vi "Model Initial Values - Get Number of Inports.vi"(8 "error in (no error)":errorcluster, 11 "ID in":T1 format="%.0x") -> (0 "error out":errorcluster, 1 "GetInportTime":u32, 2 "size(s)":i32, 3 "ID out":T1 format="%.0x", 4 "Numeric":i32)   [LabVIEW 2011, in "Model Initial Values Custom Device.lvlib"]
uses:
  Model Initial Values Custom Device.lvlib
  NationalInstruments.VeriStand.SystemDefinitionAPI
  <vilib>/NI Veristand/Custom Device Offline API/Custom Device Offline API.lvlib
  <vilib>/NI Veristand/Custom Device API/Custom Device Item Ref.ctl
  <vilib>/NI Veristand/Custom Device API/Custom Device API.lvlib
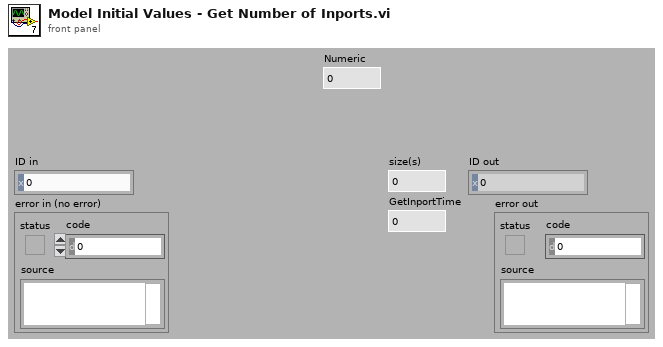
[diagram p1: front panel]
types:
  T1 = typedef "Custom Device API.lvlib/Custom Device Item Ref.ctl" = u64
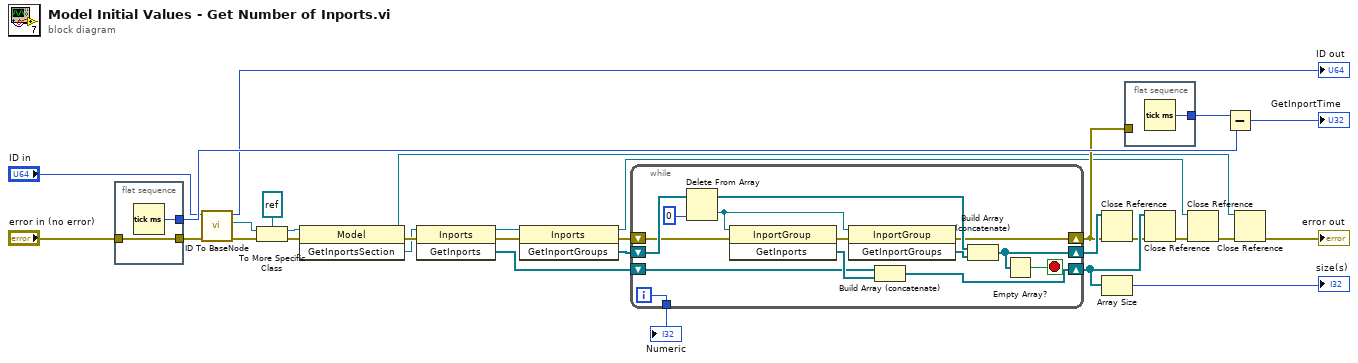
[diagram p0: block diagram]
diagram:
  n1 = flat-sequence {
    tunnel: [w32] -> w23
    tunnel: "error in (no error)" -> [w31]
    tunnel: [w31] -> w16
    frame #0 {
      n2 = Tick Count (ms)() -> (millisecond timer value=w32:u32)
    }
  }
  n3 = call <vilib>:"ID To BaseNode.vi"("error in (no error)"=w16, "ID in"="ID in") -> ("error out"=w28:errorcluster, "BaseNode"=w30:refnum<k24>, "ID out"=→"ID out":u64)  [unwired: 7 in]
  n4 = To More Specific Class(target class=refnum<k24> refnum ("BaseNodeType"), reference=w30, error in=w28) -> (specific class reference=w26:refnum<k24>, error out=w18:errorcluster)
  n5 = invoke class="Model" method="GetInportsSection"(reference=w26, error in=w18) -> (reference out=w2:refnum<k24>, error out=w25:errorcluster, "GetInportsSection"=w15:refnum<k24>)  [unwired: 1 in]
  n6 = invoke class="Inports" method="GetInports"(reference=w15, error in=w25) -> (reference out=w6:refnum<k24>, error out=w12:errorcluster, "GetInports"=w13:refnum<k24>[])  [unwired: 1 in]
  n7 = invoke class="Inports" method="GetInportGroups"(reference=w6, error in=w12) -> (reference out=w5:refnum<k24>, error out=w11:errorcluster, "GetInportGroups"=w14:refnum<k24>[])  [unwired: 1 in]
  n8 = while {
    shift-right: [w37] -> w9
    shift-left: w14 -> [w46]
    shift-right: [w40] -> w10
    shift-left: w13 -> [w39]
    shift-right: [w34] -> w7
    shift-left: w11 -> [w36]
    tunnel: [w33] -> w1
    i -> [w33]
    stop <- w38 stop-if-true
    n9 = Delete From Array(array=w46, index=0) -> (deleted portion=w42:refnum<k24>, array with subset deleted=w44:refnum<k24>[])  [unwired: 1 in]
    n10 = invoke class="InportGroup" method="GetInports"(reference=w42, error in=w36) -> (error out=w35:errorcluster, "GetInports"=w41:refnum<k24>[])  [unwired: 1 in, 1 out]
    n11 = invoke class="InportGroup" method="GetInportGroups"(reference=w42, error in=w35) -> (error out=w34:errorcluster, "GetInportGroups"=w43:refnum<k24>[])  [unwired: 1 in, 1 out]
    n12 = Build Array (concatenate)(w39, w41) -> (w40:refnum<k24>[])
    n13 = Build Array (concatenate)(w44, w43) -> (w37:refnum<k24>[])
    n14 = Empty Array?(array=w37) -> (empty?=w38:bool)
  }
  "Numeric" <- w1
  n15 = Close Reference(reference=w9, error in (no error)=w7) -> (error out=w8:errorcluster)
  n16 = Array Size(array=w10) -> (size(s)=→"size(s)":i32)
  n17 = flat-sequence {
    tunnel: [w47] -> w24
    tunnel: w7 -> [_]
    frame #0 {
      n18 = Tick Count (ms)() -> (millisecond timer value=w47:u32)
    }
  }
  n19 = Close Reference(reference=w10, error in (no error)=w8) -> (error out=w19:errorcluster)
  n20 = Close Reference(reference=w5, error in (no error)=w19) -> (error out=w4:errorcluster)
  n21 = Subtract(x=w24, y=w23) -> (x-y=→"GetInportTime":u32)
  n22 = Close Reference(reference=w2, error in (no error)=w4) -> (error out=→"error out":errorcluster)
